vi "Teleop.vi"(10 "Match Info":T1={"Autonomous Elapsed Seconds"=0.0, "TeleOp Elapsed Seconds"=0.0, "Disabled Elapsed Seconds"=0.0, "Visited Autonomous"=FALSE, "Visited TeleOp"=FALSE, "Visited Disabled"=FALSE, "Autonomous Settings"={"Autonomous Style"=enum."Independent", "VI Refnum"=refnum}}, 11 "Call Context":T2) -> ()   [LabVIEW 2020]
doc: "This VI is called for each TeleOp packet received from the DS where the robot is not disabled. It is often used to read from the joysticks and update I/O or to update setpoints for timed control loops. It should complete and return within 20 milliseconds or it may miss DS packets."
uses:
  <vilib>/Rock Robotics/WPI/DriverStation/WPI_DriverStationDerivedRobotMode.ctl
  <vilib>/Rock Robotics/WPI/DriverStation/WPI_DriverStationMatch Info.ctl
  <vilib>/Rock Robotics/WPI/Solenoid/WPI_SolenoidValue.ctl
  <vilib>/Rock Robotics/WPI/ThirdParty/REV Robotics/REVLib/Typedef/Spark MAX Control Type.ctl
  Robot Global Data.vi
  <vilib>/Rock Robotics/WPI/Utilities/WPI_GetSetVariantRefNum.vi
  <vilib>/Rock Robotics/WPI/Solenoid/WPI_SolenoidSetEnum.vi
  <vilib>/Rock Robotics/Network Tables/NT Read Boolean.vi
  <vilib>/Rock Robotics/Network Tables/NT Read Number.vi
panel:
  out "Gripper Controlled by Driver?":bool
  out "Sample Slider 0":dbl(slide) scale=0.0..5.0
  out "Sample Boolean 1":bool
  out "Sample Boolean 0":bool
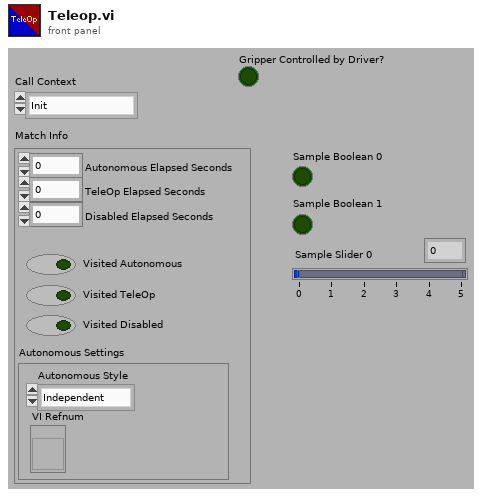
[diagram p1: front panel]
types:
  T1 = typedef "WPI_DriverStationMatch Info.ctl" = cluster{"Autonomous Elapsed Seconds":dbl, "TeleOp Elapsed Seconds":dbl, "Disabled Elapsed Seconds":dbl, "Visited Autonomous":bool, "Visited TeleOp":bool, "Visited Disabled":bool, "Autonomous Settings":cluster{"Autonomous Style":enum16{"Iterative", "Independent"}, "VI Refnum":refnum<vi>}}
  T2 = typedef "WPI_DriverStationDerivedRobotMode.ctl" = enum16{"Init", "Execute", "Stop"}
  T3 = typedef "WPI_SolenoidValue.ctl" = enum16{"Off", "On", "Forward", "Reverse"}
  T4 = enum16{"Manual", "High Cone", "High Cube", "Mid Cone", "Mid Cube", "Intake", "Cube Handoff", "Cone Handoff", "Stow"}
  T5 = typedef "Joystick_Controls.ctl" = cluster{"Pilot Left Joystick X":dbl, "Pilot Left Joystick Y":dbl, "Pilot X Button":bool, "Pilot Circle Button":bool, "Pilot Square Button":bool, "Pilot Triangle Button":bool, "Pilot Left Bumper":bool, "Pilot Right Bumper":bool, "Pilot Share Button":bool, "Pilot Options Button":bool, "Pilot Left Joystick Press":bool, "Pilot Right Joystick Press":bool, "Pilot Left Trigger":dbl, "Pilot Right Joystick X":dbl, "Pilot Right Joystick Y":dbl, "Pilot Right Trigger":dbl, "Copilot Left Joystick X":dbl, "Copilot Left Joystick Y":dbl, "Copilot X Button":bool, "Copilot Circle Button":bool, "Copilot Square Button":bool, "Copilot Triangle Button":bool, "Copilot Left Bumper":bool, "Copilot Right Bumper":bool, "Copilot Share Button":bool, "Copilot Options Button":bool, "Copilot Left Joystick Press":bool, "Copilot Right Joystick Press":bool, "Copilot Left Trigger":dbl, "Copilot Right Joystick X":dbl, "Copilot Right Joystick Y":dbl, "Copilot Right Trigger":dbl, "Pilot D-pad North":bool, "Pilot D-pad South":bool, "Pilot D-pad East":bool, "Pilot D-pad West":bool, "Pilot D-pad NE ":bool, "Pilot D-pad SE":bool, "Pilot D-pad SW":bool, "Pilot D-pad NW":bool, "CoPilot D-pad North":bool, "CoPilot D-pad South":bool, "CoPilot D-pad East":bool, "CoPilot D-pad West":bool, "CoPilot D-pad NE":bool, "CoPilot D-pad SE":bool, "CoPilot D-pad SW":bool, "CoPilot D-pad NW":bool, "Pilot Left Trigger Pressed":bool, "Pilot Right Trigger Pressed":bool, "CoPilot Left Trigger Pressed":bool, "CoPilot Right Trigger Pressed":bool, "Pilot Left Trigger Firmly":bool, "Pilot Right Trigger Firmly":bool, "Pilot Touchpad":bool, "Pilot PS Button":bool, "CoPilot Left Trigger Firmly":bool, "CoPilot Right Trigger Firmly":bool, "CoPilot Touchpad":bool, "CoPilot PS Button":bool}
  T6 = typedef "WPI_MotorControlDeviceRef.ctl" = cluster{"DeviceStatus":errorcluster, "Type":T7, "PWM":cluster{"PWM Channel":T8, "DeadBand":T9}, "CAN":cluster{"Device Number":u8, "SetOutput VI Ref":variant, "GetOutput VI Ref":variant, "Enable VI Ref":variant, "Disable VI Ref":variant, "Data":variant}, "Invert":bool, "DIO PWM":cluster{"PWM \"Enable\" Channel":T8, "DIOChannel":T10, "PWM Rate":dbl}}
  T7 = typedef "WPI_MotorControlType.ctl" = enum16{"PWM", "CAN", "DIO PWM"}
  T8 = typedef "FPGA_DIOPWMChannel.ctl" = enum8{"PWM 0", "PWM 1", "PWM 2", "PWM 3", "PWM 4", "PWM 5", "PWM 6", "PWM 7", "PWM 8", "PWM 9", "PWM MXP 0", "PWM MXP 1", "PWM MXP 2", "PWM MXP 3", "PWM MXP 4", "PWM MXP 5", "PWM MXP 6", "PWM MXP 7", "PWM MXP 8", "PWM MXP 9", "Invalid"}
  T9 = typedef "WPI_PWMDeadband.ctl" = cluster{"Name":string, "maxPositivePwm":i32, "minPositivePwm":i32, "centerPwm":i32, "maxNegativePwm":i32, "minNegativePwm":i32, "angularRange":u16}
  T10 = typedef "FPGA_DIOChannel.ctl" = enum8{"DIO 0", "DIO 1", "DIO 2", "DIO 3", "DIO 4", "DIO 5", "DIO 6", "DIO 7", "DIO 8", "DIO 9", "DIO MXP 0", "DIO MXP 1", "DIO MXP 2", "DIO MXP 3", "DIO MXP 4", "DIO MXP 5", "DIO MXP 6", "DIO MXP 7", "DIO MXP 8", "DIO MXP 9", "DIO MXP 10", "DIO MXP 11", "DIO MXP 12", "DIO MXP 13", "DIO MXP 14", "DIO MXP 15", "SPI Port CS1", "SPI Port CS2", "SPI Port CS3", "SPI Port MISO", "SPI Port MOSI", "Invalid"}
  T11 = typedef "Spark MAX Control Type.ctl" = enum16{"Percent VBus", "Voltage", "Velocity", "Position", "Smart Motion", "Current", "Smart Velocity"}
  T12 = typedef "WPI_SolenoidDevRef.ctl" = cluster{"DevStatus":errorcluster, "Pneumatics Control Module":u8, "Forward Solenoid Channel":T13, "Reverse Solenoid Channel":T13}
  T13 = typedef "WPI_SolenoidChannel.ctl" = enum8{"Solenoid 0", "Solenoid 1", "Solenoid 2", "Solenoid 3", "Solenoid 4", "Solenoid 5", "Solenoid 6", "Solenoid 7", "Solenoid 8", "Solenoid 9", "Solenoid 10", "Solenoid 11", "Solenoid 12", "Solenoid 13", "Solenoid 14", "Solenoid 15", "Invalid"}
  T14 = typedef "WPI_RobotDriveDevRef.ctl" = cluster{"DevStatus":errorcluster, "Motors[]":T6[], "Square Inputs":bool, "Max Output":dbl}
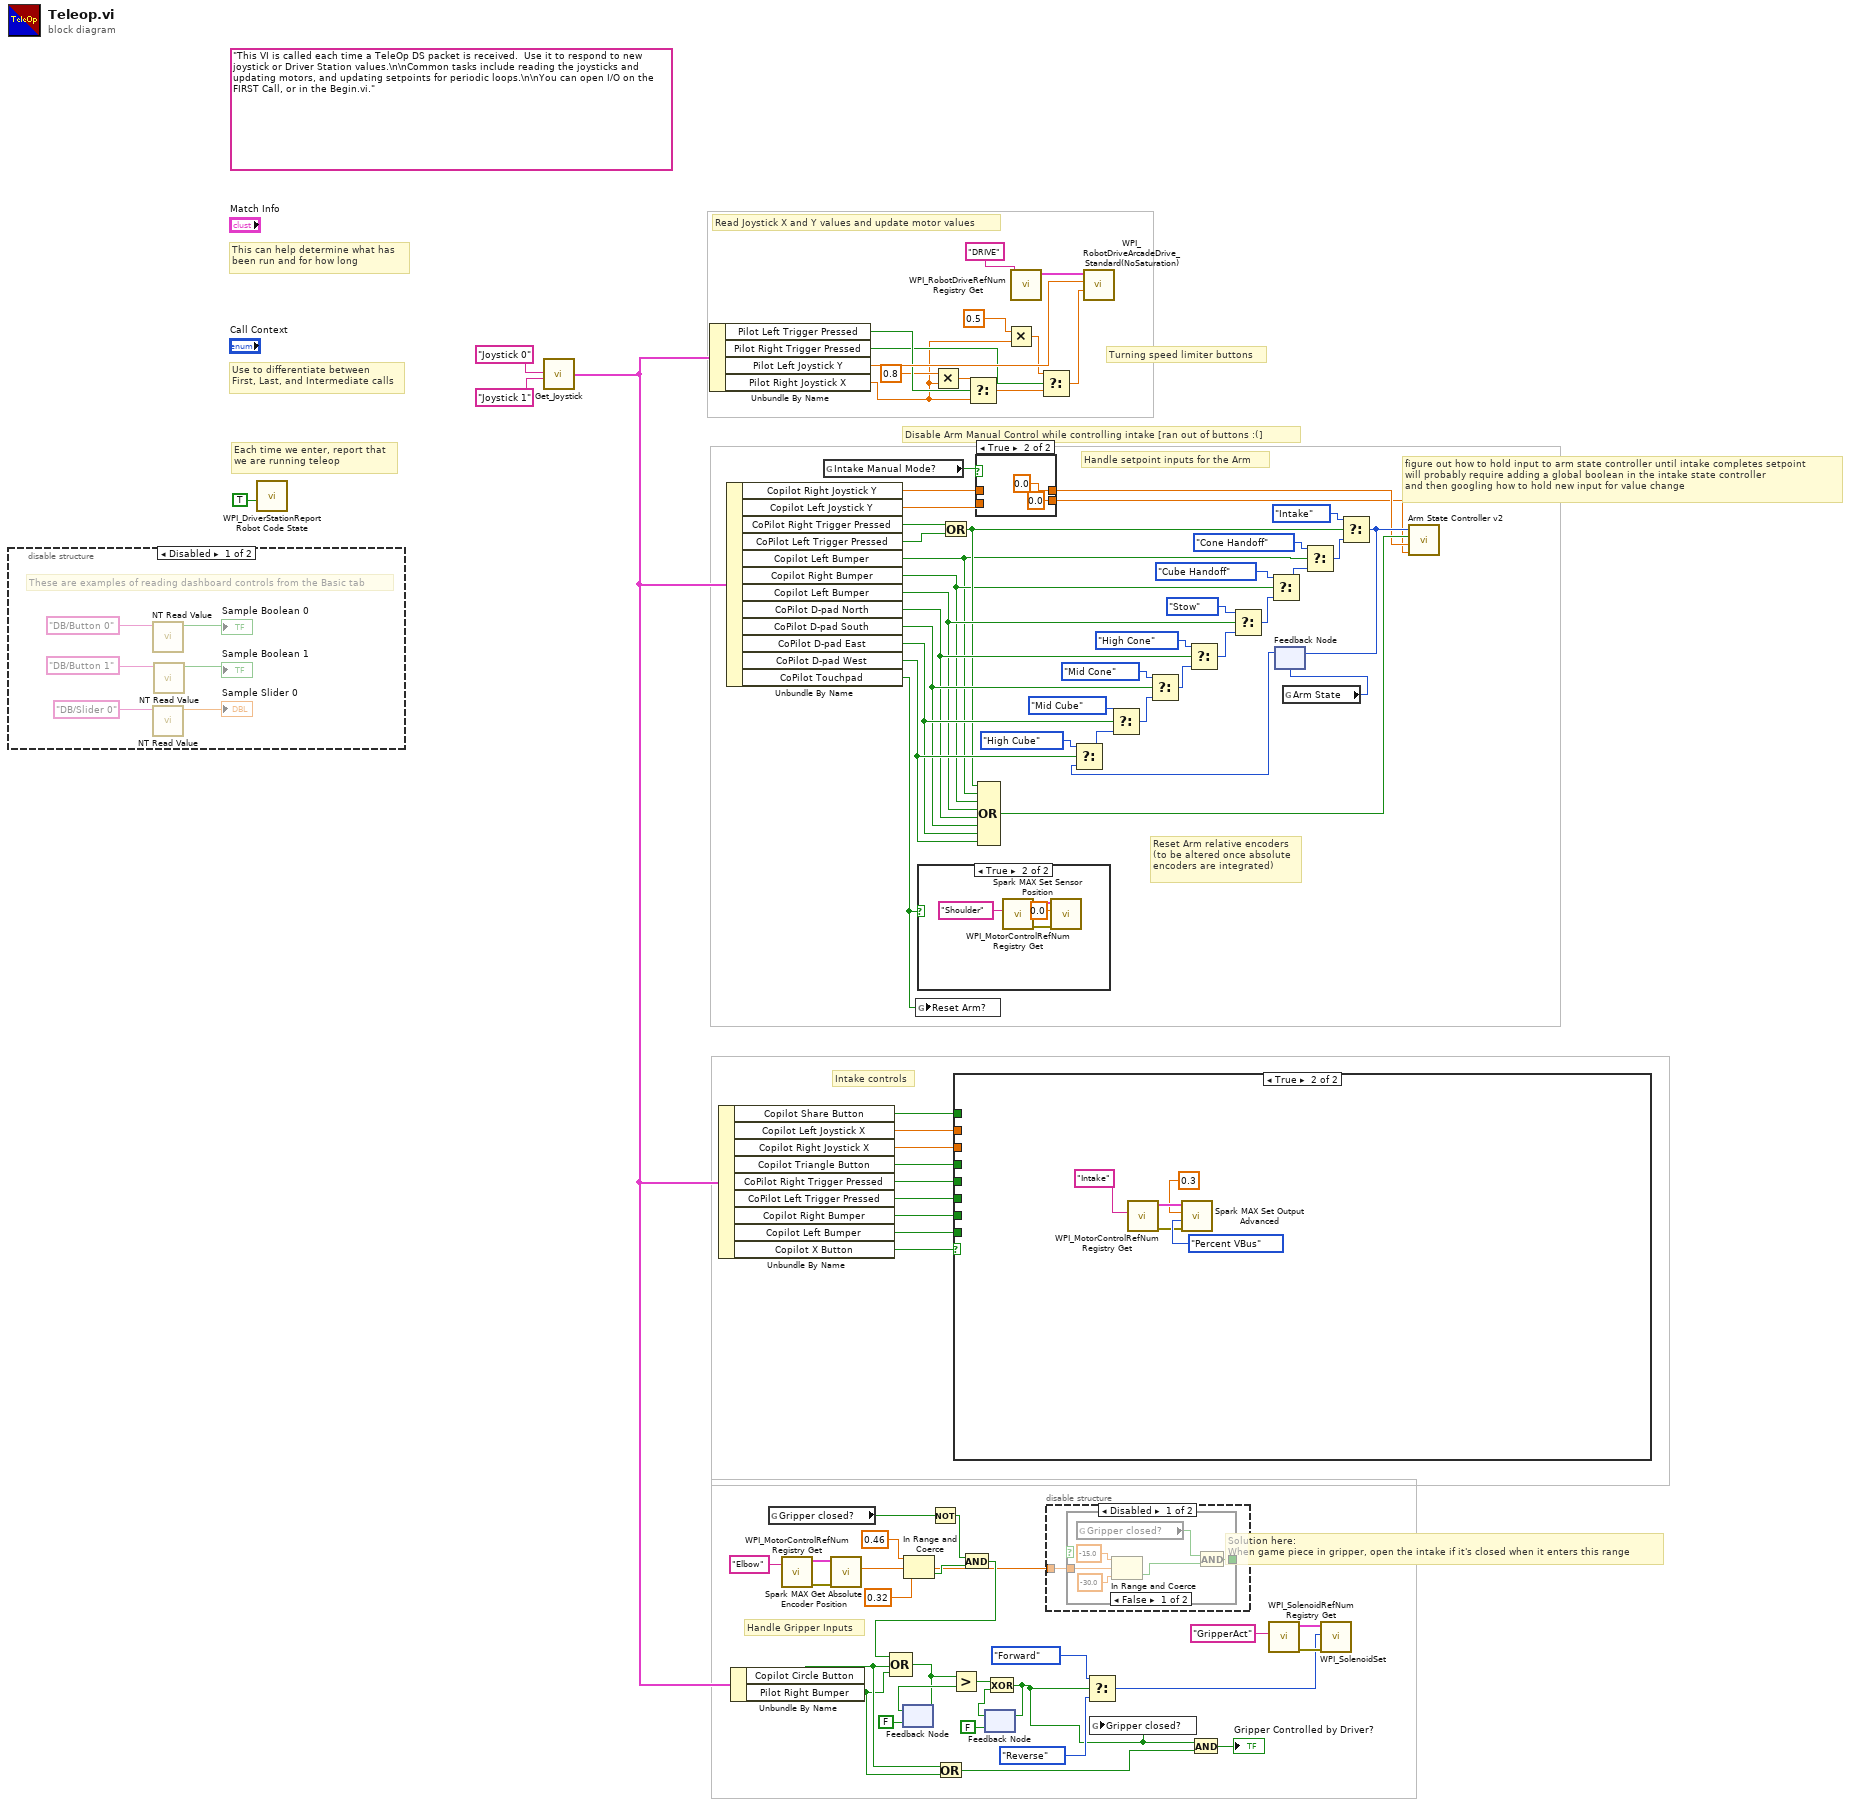
[diagram p0: block diagram]
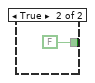
[diagram p2: hidden frame]
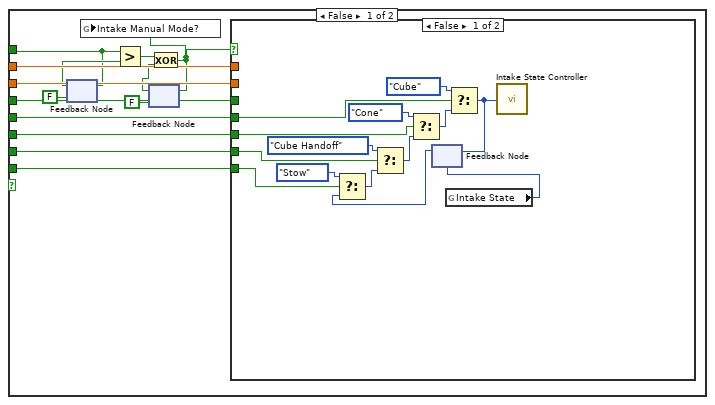
[diagram p6: hidden frame]
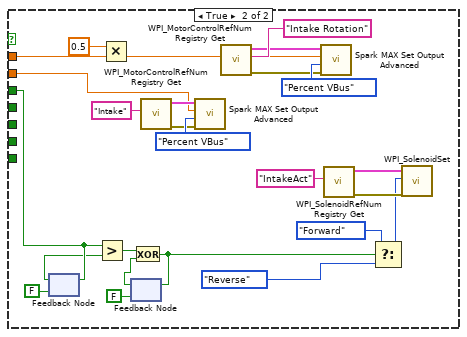
[diagram p7: hidden frame]
diagram:
  (unwired) "This VI is called each time a TeleOp DS packet is received.  Use it to respond to new joystick or Driver Station values.\n\nCommon tasks include reading the joysticks and updating motors, and updating setpoints for periodic loops.\n\nYou can open I/O on the FIRST Call, or in the Begin.vi."
  # "figure out how to hold input to arm state controller until intake completes setpoint\nwill probably require adding a global boolean in the intake state controller\nand then googling how to hold new input for value change"
  # "Solution here:\nWhen game piece in gripper, open the intake if it's closed when it enters this range"
  # "Turning speed limiter buttons"
  # "Reset Arm relative encoders\n(to be altered once absolute\nencoders are integrated)"
  # "Disable Arm Manual Control while controlling intake [ran out of buttons :(]"
  # "Handle Gripper Inputs"
  # "Handle setpoint inputs for the Arm"
  # "Intake controls"
  # "Each time we enter, report that\nwe are running teleop"
  # "Use to differentiate between\nFirst, Last, and Intermediate calls"
  # "This can help determine what has\nbeen run and for how long"
  # "Read Joystick X and Y values and update motor values"
  n1 = disable-structure shown="Disabled" {
    frame Disabled {
      # "These are examples of reading dashboard controls from the Basic tab"
      n2 = call-poly <vilib>:"NT Read Value.vi"("name"="DB/Button 0" ("refnum name")) -> ("value"=→"Sample Boolean 0":bool)  [unwired: 8 in, 2 out]
      n3 = call-poly <vilib>:"NT Read Value.vi"("name"="DB/Slider 0" ("refnum name")) -> ("value"=→"Sample Slider 0":dbl)  [unwired: 8 in, 2 out]
      n4 = call-poly <vilib>:"NT Read Value.vi"("name"="DB/Button 1" ("refnum name")) -> ("value"=→"Sample Boolean 1":bool)  [unwired: 8 in, 2 out]
    }
    frame Enabled {
    }
  }
  n5 = call <vilib>:"WPI_DriverStationReport Robot Code State.vi"("TeleOp"=TRUE ("Autonomous")) -> ()  [unwired: 10 in, 1 out]
  n6 = call "Get_Joystick.vi"("Joystick_One"="Joystick 0" ("refnum name"), "Joystick_Two"="Joystick 1") -> ("Joystick_Out"=w82:T5)  [unwired: 5 in]
  n7 = Unbundle By Name(w82) -> ("Pilot Left Trigger Pressed"=w80:bool, "Pilot Right Trigger Pressed"=w76:bool, "Pilot Left Joystick Y"=w81:dbl, "Pilot Right Joystick X"=w74:dbl)
  n8 = Unbundle By Name(w82) -> ("Copilot Share Button"=w12:bool, "Copilot Left Joystick X"=w67:dbl, "Copilot Right Joystick X"=w65:dbl, "Copilot Triangle Button"=w66:bool, "CoPilot Right Trigger Pressed"=w68:bool, "CoPilot Left Trigger Pressed"=w69:bool, "Copilot Right Bumper"=w70:bool, "Copilot Left Bumper"=w71:bool, "Copilot X Button"=w64:bool)
  n9 = Unbundle By Name(w82) -> ("Copilot Right Joystick Y"=w10:dbl, "Copilot Left Joystick Y"=w8:dbl, "CoPilot Right Trigger Pressed"=w48:bool, "CoPilot Left Trigger Pressed"=w47:bool, "Copilot Left Bumper"=w36:bool, "Copilot Right Bumper"=w37:bool, "Copilot Left Bumper"=w42:bool, "CoPilot D-pad North"=w43:bool, "CoPilot D-pad South"=w44:bool, "CoPilot D-pad East"=w45:bool, "CoPilot D-pad West"=w46:bool, "CoPilot Touchpad"=w39:bool)
  n10 = Unbundle By Name(w82) -> ("Copilot Circle Button"=w3:bool, "Pilot Right Bumper"=w2:bool)
  n11 = global read "Robot Global Data.vi" "Gripper closed?"() -> (w16:bool)
  n12 = call <vilib>:"WPI_MotorControlRefNum Registry Get.vi"("refnum name"="Elbow") -> ("error out"=w20:errorcluster, "MotorControlDevRef"=w19:T6)  [unwired: 9 in]
  n13 = global read "Robot Global Data.vi" "Intake Manual Mode?"() -> (w11:bool)
  n14 = call <vilib>:"Spark MAX Get Absolute Encoder Position.vi"("error in (no error)"=w20, "MotorControlDeviceRef in"=w19) -> ("Position"=w6:dbl)  [unwired: 6 in, 3 out]
  n15 = feedback #1(FALSE ("Copilot X Button")) -> (w30:bool)
  n16 = In Range and Coerce(upper limit=0.46, x=w6, lower limit=0.32) -> (In Range?=w15:bool)  [unwired: 1 out]
  n17 = global write "Robot Global Data.vi" "Reset Arm?"(w39) -> ()
  n18 = case shown="True" w39 {
    frame False {
    }
    frame True {
      n19 = call <vilib>:"WPI_MotorControlRefNum Registry Get.vi"("refnum name"="Shoulder") -> ("error out"=w97:errorcluster, "MotorControlDevRef"=w96:T6)  [unwired: 9 in]
      n20 = call <vilib>:"Spark MAX Set Sensor Position.vi"("error in"=w97, "Position"=0.0, "MotorControlDeviceRef"=w96) -> ()  [unwired: 7 in, 2 out]
    }
  }
  n21 = Not(x=w16) -> (.not. x?=w14:bool)
  n22 = Multiply(x=0.8, y=w74) -> (x*y=w79:dbl)
  n23 = Or(x=w3, y=w2) -> (x .or. y?=w4:bool)
  n24 = Or(x=w48, y=w47) -> (x .or. y?=w41:bool)
  n25 = case shown="True" w64 {
    tunnel: w71 -> [w111 _]
    tunnel: w70 -> [w110 _]
    tunnel: w69 -> [w109 _]
    tunnel: w68 -> [w108 _]
    tunnel: w67 -> [w107 _]
    tunnel: w66 -> [w106 _]
    tunnel: w65 -> [w105 _]
    tunnel: w12 -> [w99 _]
    frame False {
      n26 = feedback #2(FALSE ("Copilot X Button")) -> (w104:bool)
      n27 = feedback-in #2(w99) -> ()
      n28 = Greater?(x=w99, y=w104) -> (0:w102:bool)
      n29 = feedback #3(FALSE) -> (w101:bool)
      n30 = Exclusive Or(1:w101, 2:w102) -> (0:w98:bool)
      n31 = global write "Robot Global Data.vi" "Intake Manual Mode?"(w98) -> ()
      n32 = feedback-in #3(w98) -> ()
      n33 = case shown="False" w98 {
        tunnel: w111 -> [w125 _]
        tunnel: w110 -> [w124 _]
        tunnel: w109 -> [w123 _]
        tunnel: w108 -> [w122 _]
        tunnel: w107 -> [_ w141]
        tunnel: w106 -> [_ w138]
        tunnel: w105 -> [_ w146]
        frame False {
          n34 = global read "Robot Global Data.vi" "Intake State"() -> (w112:enum16{"Cone", "Cube", "Cube Handoff", "Stow"})
          n35 = feedback #4(w112) -> (w114:enum16{"Cone", "Cube", "Cube Handoff", "Stow"})
          n36 = Select(t=enum16{"Cone", "Cube", "Cube Handoff", "Stow"}."Stow" ("Intake State"), s=w125, f=w114) -> (s? t:f=w120:enum16{"Cone", "Cube", "Cube Handoff", "Stow"})
          n37 = Select(t=enum16{"Cone", "Cube", "Cube Handoff", "Stow"}."Cube Handoff" ("Intake State"), s=w124, f=w120) -> (s? t:f=w117:enum16{"Cone", "Cube", "Cube Handoff", "Stow"})
          n38 = Select(t=enum16{"Cone", "Cube", "Cube Handoff", "Stow"}."Cone" ("Intake State"), s=w123, f=w117) -> (s? t:f=w115:enum16{"Cone", "Cube", "Cube Handoff", "Stow"})
          n39 = Select(t=enum16{"Cone", "Cube", "Cube Handoff", "Stow"}."Cube" ("Intake State"), s=w122, f=w115) -> (s? t:f=w113:enum16{"Cone", "Cube", "Cube Handoff", "Stow"})
          n40 = feedback-in #4(w113) -> ()
          n41 = call "Intake State Controller.vi"("Intake State"=w113) -> ()
        }
        frame True {
          n42 = feedback-in #5(w138) -> ()
          n43 = feedback #5(FALSE ("Copilot X Button")) -> (w137:bool)
          n44 = Greater?(x=w138, y=w137) -> (0:w135:bool)
          n45 = Multiply(x=0.5, y=w141) -> (x*y=w140:dbl)
          n46 = feedback #6(FALSE) -> (w134:bool)
          n47 = Exclusive Or(1:w134, 2:w135) -> (0:w131:bool)
          n48 = feedback-in #6(w131) -> ()
          n49 = call <vilib>:"WPI_MotorControlRefNum Registry Get.vi"("refnum name"="Intake") -> ("error out"=w147:errorcluster, "MotorControlDevRef"=w148:T6)  [unwired: 9 in]
          n50 = call <vilib>:"Spark MAX Set Output Advanced.vi"("error in (no error)"=w147, "Control Mode"=Spark_MAX_Control_Type."Percent VBus", "Setpoint"=w146, "MotorControlDevRef"=w148) -> ()  [unwired: 6 in, 2 out]
          n51 = call <vilib>:"WPI_MotorControlRefNum Registry Get.vi"("refnum name"="Intake Rotation") -> ("error out"=w142:errorcluster, "MotorControlDevRef"=w143:T6)  [unwired: 9 in]
          n52 = call <vilib>:"Spark MAX Set Output Advanced.vi"("error in (no error)"=w142, "Control Mode"=Spark_MAX_Control_Type."Percent VBus", "Setpoint"=w140, "MotorControlDevRef"=w143) -> ()  [unwired: 6 in, 2 out]
          n53 = call <vilib>:"WPI_SolenoidRefNum Registry Get.vi"("refnum name"="IntakeAct") -> ("error out"=w128:errorcluster, "SolenoidDevRef"=w127:T12)  [unwired: 9 in]
          n54 = Select(t=WPI_SolenoidValue."Forward" ("Value"), s=w131, f=WPI_SolenoidValue."Reverse") -> (s? t:f=w126:T3)
          n55 = call-poly <vilib>:"WPI_SolenoidSet.vi"("error in (no error)"=w128, "Value"=w126, "SolenoidDevRef"=w127) -> ()  [unwired: 7 in, 2 out]
        }
      }
    }
    frame True {
      n56 = call <vilib>:"WPI_MotorControlRefNum Registry Get.vi"("refnum name"="Intake") -> ("error out"=w152:errorcluster, "MotorControlDevRef"=w153:T6)  [unwired: 9 in]
      n57 = call <vilib>:"Spark MAX Set Output Advanced.vi"("error in (no error)"=w152, "Control Mode"=Spark_MAX_Control_Type."Percent VBus", "Setpoint"=0.3, "MotorControlDevRef"=w153) -> ()  [unwired: 6 in, 2 out]
    }
  }
  n58 = And(x=w14, y=w15) -> (x .and. y?=w13:bool)
  n59 = Compound Arithmetic op=OR(w13, w3, w2) -> (w22:bool)
  n60 = feedback-in #1(w22) -> ()
  n61 = Greater?(x=w22, y=w30) -> (0:w28:bool)
  n62 = Select(t=w79, s=w80, f=w74) -> (s? t:f=w77:dbl)
  n63 = case shown="True" w11 {
    tunnel: w10 -> [w157 _]
    tunnel: [w157 0.0 ("Copilot Right Joystick Y")] -> w9
    tunnel: w8 -> [w156 _]
    tunnel: [w156 0.0 ("Copilot Left Joystick Y")] -> w7
    frame False {
    }
    frame True {
    }
  }
  n64 = Compound Arithmetic op=OR(w41, w36, w37, w42, w43, w44, w45, w46) -> (w35:bool)
  n65 = feedback #7(FALSE) -> (w27:bool)
  n66 = Exclusive Or(1:w27, 2:w28) -> (0:w1:bool)
  n67 = feedback-in #7(w1) -> ()
  n68 = Multiply(x=0.5, y=w74) -> (x*y=w75:dbl)
  n69 = call <vilib>:"WPI_RobotDriveRefNum Registry Get.vi"("refnum name"="DRIVE") -> ("RobotDriveDevRef"=w86:T14)  [unwired: 1 in, 9 out]
  n70 = Select(t=w75, s=w76, f=w77) -> (s? t:f=w72:dbl)
  n71 = disable-structure shown="Disabled" {
    disable-tunnel: w6 -> [w160 _]
    frame Disabled {
      n72 = case shown="False" {
        selector: _ -> [_ _]
        tunnel: w160 -> [w166 _]
        tunnel: [w161 FALSE] -> _
        frame False {
          n73 = global read "Robot Global Data.vi" "Gripper closed?"() -> (w162:bool)
          n74 = In Range and Coerce(upper limit=-15.0, x=w166, lower limit=-30.0) -> (In Range?=w163:bool)  [unwired: 1 out]
          n75 = And(x=w162, y=w163) -> (x .and. y?=w161:bool)
        }
        frame True {
        }
      }
    }
    frame Enabled {
    }
  }
  n76 = call <vilib>:"WPI_RobotDriveArcadeDrive_Standard(NoSaturation).vi"("Y axis value"=w72, "X axis value"=w81, "RobotDriveDevRef"=w86) -> ()  [unwired: 1 in, 8 out]
  n77 = Select(t=WPI_SolenoidValue."Forward" ("f"), s=w1, f=WPI_SolenoidValue."Reverse") -> (s? t:f=w23:T3)
  n78 = global write "Robot Global Data.vi" "Gripper closed?"(w1) -> ()
  n79 = And(x=w1, y=w4) -> (x .and. y?=→"Gripper Controlled by Driver?":bool)
  n80 = call <vilib>:"WPI_SolenoidRefNum Registry Get.vi"("refnum name"="GripperAct") -> ("error out"=w34:errorcluster, "SolenoidDevRef"=w33:T12)  [unwired: 9 in]
  n81 = global read "Robot Global Data.vi" "Arm State"() -> (w38:T4)
  n82 = feedback #8(w38) -> (w40:T4)
  n83 = Select(t=T4."High Cube" ("Target Arm State"), s=w46, f=w40) -> (s? t:f=w61:T4)
  n84 = Select(t=T4."Mid Cube" ("Target Arm State"), s=w45, f=w61) -> (s? t:f=w59:T4)
  n85 = Select(t=T4."Mid Cone" ("Target Arm State"), s=w44, f=w59) -> (s? t:f=w57:T4)
  n86 = Select(t=T4."High Cone" ("Target Arm State"), s=w43, f=w57) -> (s? t:f=w55:T4)
  n87 = Select(t=T4."Stow" ("Target Arm State"), s=w42, f=w55) -> (s? t:f=w53:T4)
  n88 = Select(t=T4."Cube Handoff" ("Target Arm State"), s=w37, f=w53) -> (s? t:f=w51:T4)
  n89 = Select(t=T4."Cone Handoff" ("Target Arm State"), s=w36, f=w51) -> (s? t:f=w49:T4)
  n90 = call-poly <vilib>:"WPI_SolenoidSet.vi"("error in (no error)"=w34, "Value"=w23, "SolenoidDevRef"=w33) -> ()  [unwired: 7 in, 2 out]
  n91 = Select(t=T4."Intake" ("Target Arm State"), s=w41, f=w49) -> (s? t:f=w31:T4)
  n92 = feedback-in #8(w31) -> ()
  n93 = call "Arm State Controller v2.vi"("Elbow Manual Power"=w7, "Shoulder Manual Power"=w9, "Setpoint Change Detected?"=w35, "Target Arm State"=w31) -> ()
